vi "_Create (Friend).vi"(8 "error in (no error)":errorcluster, 11 "ListImp in":refnum<class "ListImp.lvclass">) -> (0 "error out":errorcluster, 3 "ListImp out":refnum<class "ListImp.lvclass">)   [LabVIEW 2013, in "LapDog.Collections.v_.Lists.lvlib" / "ListImp.lvclass"]
doc: "This method is invoked when List:Create is called. It should only be called by the List class. List subclasses should use the List:CreateImplementation method, which delegates to this method."
uses:
  ListImp.lvclass
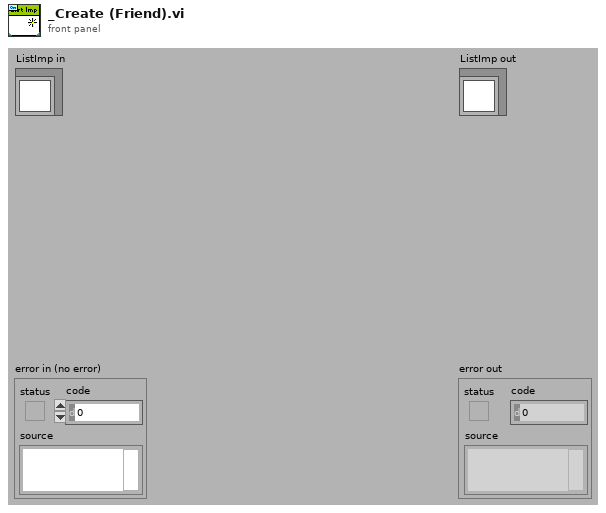
[diagram p1: front panel]
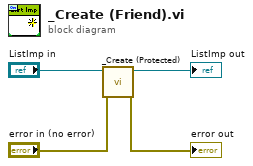
[diagram p0: block diagram]
diagram:
  n1 = call-dynamic "_Create (Protected).vi"("error in (no error)"="error in (no error)", "ListImp in"="ListImp in") -> ("error out"=→"error out":errorcluster, "ListImp out"=→"ListImp out":refnum<class "ListImp.lvclass">)  [unwired: 8 in]
